vi "UHR-Fleezers Control (host) - 11.1.vi"() -> ()   [LabVIEW 2012] (continued)
            n2044 = Unbundle By Name(w3406) -> ("Set 1"=w3405:dbl, "Set 2"=w3404:dbl)
            n2045 = Unbundle By Name(w3412) -> ("Set 1"=w3411:dbl, "Set 2"=w3410:dbl)
            n2046 = Unbundle By Name(w3409) -> ("Set 1"=w3408:bool, "Set 2"=w3407:bool)
            n2047 = Select(t=w3405, s=w3408, f=w3411) -> (s? t:f=w3403:dbl)
            n2048 = Select(t=w3404, s=w3407, f=w3410) -> (s? t:f=w3402:dbl)
            n2049 = Bundle By Name(cluster=w3412, "Set 1"=w3403, "Set 2"=w3402) -> (w3400:cluster{"Set 1":dbl, "Set 2":dbl})
            n2050 = local write "Setpoints (V)"(w3400) -> ()
            n2051 = Multiply(x=3276.7, y=w3400) -> (x*y=w3401:cluster{"Set 1":dbl, "Set 2":dbl})
            n2052 = To Word Integer(number=w3401) -> (16bit integer=w3413:cluster{"Set 1":i16, "Set 2":i16})
          }
        }
        n2053 = Unbundle By Name(w3385) -> ("Set 1"=w3384:i16, "Set 2"=w3383:i16)
        n2054 = xnode "Read/Write Control"("FPGA VI Reference In"=w3381, "error in"=w3380, "FB Setpoint Set 1"=w3384, "FB Setpoint Set 2"=w3383) -> ("error out"=w3379:errorcluster)  [unwired: 1 out]
      }
      event "Invert GI": Value Change {
        n2055 = event-data() -> ()  [unwired: 7 out]
        n2056 = xnode "Read/Write Control"("FPGA VI Reference In"=w3418, "error in"=w3416, "Invert GI"="Invert GI", "Invert GI 2"="Invert GI") -> ("error out"=w3417:errorcluster)  [unwired: 1 out]
      }
      event "Green FB Setpoint (mV)", "Green FB Gains", "Green FB On/Off", "Current When FB OFF (%)", "Green int current ON count adj": Value Change {
        n2057 = event-data() -> ()  [unwired: 7 out]
        n2058 = local read "Green FB Setpoint (mV)"() -> (w3425:dbl)
        n2059 = local read "Current When FB OFF (%)"() -> (w3428:dbl)
        n2060 = Multiply(x=w3425, y=3.2767) -> (x*y=w3424:dbl)
        n2061 = Multiply(x=w3428, y=655.35) -> (x*y=w3429:dbl)
        n2062 = To Unsigned Word Integer(number=w3429) -> (unsigned 16bit integer=w3427:u16)
        n2063 = local read "Green int current ON count adj"() -> (w3432:u32)
        n2064 = local read "Green FB Gains"() -> (w3431:T14)
        n2065 = local read "Green Laser ON/Interlacing"() -> (w3422:bool)
        n2066 = local read "Green laser mode"() -> (w3421:enum32{"Laser ON", "Laser OFF", "Interlace"})
        n2067 = local read "Green FB On/Off"() -> (w3433:bool)
        n2068 = Equal?(x=w3421, y=enum32{"Laser ON", "Laser OFF", "Interlace"}."Interlace") -> (x = y?=w3419:bool)
        n2069 = Compound Arithmetic op=AND(w3419, w3433, w3422) -> (w3423:bool)
        n2070 = xnode "Read/Write Control"("FPGA VI Reference In"=w3436, "error in"=w3435, "Green FB Setpoint"=w3424, "Green FB On/Off"=w3423, "Current Out"=w3427, "Green int current ON count adj"=w3432, "Green FB Gains"=w3431) -> ("error out"=w3434:errorcluster)  [unwired: 1 out]
      }
      event "Green laser mode", "Green Laser ON/Interlacing": Value Change {
        n2071 = event-data() -> ()  [unwired: 7 out]
        n2072 = local write "Green Laser ON/OFF"("Green Laser ON/Interlacing") -> ()
        n2073 = case shown="True" "Green Laser ON/Interlacing" {
          tunnel: "Green laser mode" -> [_ w3450]
          tunnel: [enum32{"Laser ON", "Laser OFF", "Interlace"}."Laser OFF" ("Green laser mode") w3450] -> w3439
          tunnel: [FALSE w3446] -> w3438
          frame False {
          }
          frame True {
            n2074 = local read "Green FB On/Off"() -> (w3447:bool)
            n2075 = Equal?(x=w3450, y=enum32{"Laser ON", "Laser OFF", "Interlace"}."Interlace") -> (x = y?=w3448:bool)
            n2076 = And(x=w3448, y=w3447) -> (x .and. y?=w3446:bool)
          }
        }
        n2077 = xnode "Read/Write Control"("FPGA VI Reference In"=w3443, "error in"=w3441, "Operating Mode"=w3439, "Operating Mode 2"=w3439, "Green FB On/Off"=w3438) -> ("error out"=w3442:errorcluster)  [unwired: 1 out]
      }
      event "Green Laser ON/OFF": Value Change {
        n2078 = event-data() -> ()  [unwired: 7 out]
        n2079 = property on="Green Laser ON/Interlacing" class="Bool (strict)"("Val(Sgnl)"="Green Laser ON/OFF") -> ()  [unwired: 2 in, 2 out]
      }
      event "Test ttrig": Value Change {
        n2080 = event-data() -> ()  [unwired: 7 out]
        n2081 = xnode "Read/Write Control"("FPGA VI Reference In"=w3455, "error in"=w3454, "TTrig?"=TRUE) -> ("error out"=w3453:errorcluster)  [unwired: 1 out]
      }
      event "Neg. TTrig FPGA": Value Change {
        n2082 = event-data() -> ()  [unwired: 7 out]
        n2083 = xnode "Read/Write Control"("FPGA VI Reference In"=w3459, "error in"=w3458, "TTrig Negate Pos"="Neg. TTrig FPGA") -> ()  [unwired: 2 out]
      }
      event "- phase (APD 1 Gate)", "+ phase (APD 1 Gate)": Value Change {
        n2084 = event-data() -> ()  [unwired: 7 out]
        n2085 = local read "Phase Adj. (APD 1 Gate)"() -> (w3460:i16)
        n2086 = Negate(x=w3460) -> (-x=w3468:i16)
        n2087 = Select(t=w3468, s="- phase (APD 1 Gate)", f=w3460) -> (s? t:f=w3467:i16)
        n2088 = Or(x="- phase (APD 1 Gate)", y="+ phase (APD 1 Gate)") -> (x .or. y?=w3463:bool)
        n2089 = xnode "Read/Write Control"("FPGA VI Reference In"=w3470, "error in"=w3469, "Phase count adjustment (APD 1 Gate)"=w3467) -> ("FPGA VI Reference Out"=w3465:T19, "error out"=w3466:errorcluster)
        n2090 = xnode "Read/Write Control"("FPGA VI Reference In"=w3465, "error in"=w3466, "+ phase (APD 1 Gate)"=w3463) -> ("error out"=w3464:errorcluster)  [unwired: 1 out]
      }
      event "+ phase (APD 2 Gate)", "- phase (APD 2 Gate)": Value Change {
        n2091 = event-data() -> ()  [unwired: 7 out]
        n2092 = local read "Phase Adj. (APD 2 Gate)"() -> (w3471:i16)
        n2093 = Negate(x=w3471) -> (-x=w3479:i16)
        n2094 = Select(t=w3479, s="- phase (APD 2 Gate)", f=w3471) -> (s? t:f=w3478:i16)
        n2095 = Or(x="- phase (APD 2 Gate)", y="+ phase (APD 2 Gate)") -> (x .or. y?=w3474:bool)
        n2096 = xnode "Read/Write Control"("FPGA VI Reference In"=w3481, "error in"=w3480, "Phase count adjustment (APD 2 Gate)"=w3478) -> ("FPGA VI Reference Out"=w3476:T19, "error out"=w3477:errorcluster)
        n2097 = xnode "Read/Write Control"("FPGA VI Reference In"=w3476, "error in"=w3477, "+ phase (APD 2 Gate)"=w3474) -> ("error out"=w3475:errorcluster)  [unwired: 1 out]
      }
      event "Phase Adj. (APD Acq)", "+ phase (APD Acq)", "- phase (APD Acq)": Value Change {
        n2098 = event-data() -> ()  [unwired: 7 out]
        n2099 = local read "Phase Adj. (APD Acq)"() -> (w3484:i16)
        n2100 = Negate(x=w3484) -> (-x=w3490:i16)
        n2101 = Select(t=w3490, s="+ phase (APD Acq)", f=w3484) -> (s? t:f=w3489:i16)
        n2102 = Or(x="+ phase (APD Acq)", y="- phase (APD Acq)") -> (x .or. y?=w3485:bool)
        n2103 = xnode "Read/Write Control"("FPGA VI Reference In"=w3492, "error in"=w3491, "Phase Count Adjustment (APD Acq)"=w3489) -> ("FPGA VI Reference Out"=w3487:T19, "error out"=w3488:errorcluster)
        n2104 = xnode "Read/Write Control"("FPGA VI Reference In"=w3487, "error in"=w3488, "+ phase (APD Acq)"=w3485) -> ("error out"=w3486:errorcluster)  [unwired: 1 out]
      }
      event "Phase adj. (GI)", "+ phase (GI)", "- phase (GI)": Value Change {
        n2105 = event-data() -> ()  [unwired: 7 out]
        n2106 = Negate(x="Phase adj. (GI)") -> (-x=w3501:i16)
        n2107 = Select(t=w3501, s="+ phase (GI)", f="Phase adj. (GI)") -> (s? t:f=w3500:i16)
        n2108 = Or(x="+ phase (GI)", y="- phase (GI)") -> (x .or. y?=w3496:bool)
        n2109 = xnode "Read/Write Control"("FPGA VI Reference In"=w3503, "error in"=w3502, "Phase count adjustment (GI)"=w3500) -> ("FPGA VI Reference Out"=w3498:T19, "error out"=w3499:errorcluster)
        n2110 = xnode "Read/Write Control"("FPGA VI Reference In"=w3498, "error in"=w3499, "+ phase (GI)"=w3496) -> ("error out"=w3497:errorcluster)  [unwired: 1 out]
      }
      event "Phase adj. (GI) 2", "+ phase (GI) 2", "- phase (GI) 2": Value Change {
        n2111 = event-data() -> ()  [unwired: 7 out]
        n2112 = Negate(x="Phase adj. (GI) 2") -> (-x=w3512:i16)
        n2113 = Select(t=w3512, s="+ phase (GI) 2", f="Phase adj. (GI) 2") -> (s? t:f=w3511:i16)
        n2114 = Or(x="+ phase (GI) 2", y="- phase (GI) 2") -> (x .or. y?=w3507:bool)
        n2115 = xnode "Read/Write Control"("FPGA VI Reference In"=w3514, "error in"=w3513, "Phase count adjustment (GI) 2"=w3511) -> ("FPGA VI Reference Out"=w3509:T19, "error out"=w3510:errorcluster)
        n2116 = xnode "Read/Write Control"("FPGA VI Reference In"=w3509, "error in"=w3510, "+ phase (GI) 2"=w3507) -> ("error out"=w3508:errorcluster)  [unwired: 1 out]
      }
      event "Phase adj. (Green FB)", "- phase (Green FB)", "+ phase (Green FB)": Value Change {
        n2117 = event-data() -> ()  [unwired: 7 out]
        n2118 = Negate(x="Phase adj. (Green FB)") -> (-x=w3523:i16)
        n2119 = Select(t=w3523, s="+ phase (Green FB)", f="Phase adj. (Green FB)") -> (s? t:f=w3522:i16)
        n2120 = Or(x="+ phase (Green FB)", y="- phase (Green FB)") -> (x .or. y?=w3518:bool)
        n2121 = xnode "Read/Write Control"("FPGA VI Reference In"=w3525, "error in"=w3524, "Phase count adjustment (Green FB)"=w3522) -> ("FPGA VI Reference Out"=w3520:T19, "error out"=w3521:errorcluster)
        n2122 = xnode "Read/Write Control"("FPGA VI Reference In"=w3520, "error in"=w3521, "+ phase (Green FB)"=w3518) -> ("error out"=w3519:errorcluster)  [unwired: 1 out]
      }
      event "Invert APD Gate", "APD Gate ON Count", "APD Gate OFF Count", "APD Gate", "APD Integration Time (s)", "APD 1 AO Mult.", "APD 2 AO Mult.", "On one out of X cycles": Value Change {
        n2123 = event-data() -> ()  [unwired: 7 out]
        n2124 = Add(x="GI Frequency, ON count", y="GI Frequency, OFF count") -> (x+y=w3529:u32)
        n2125 = Add(x="APD Gate ON Count", y="APD Gate OFF Count") -> (x+y=w3542:u32)
        n2126 = Multiply(x="On one out of X cycles", y=w3529) -> (x*y=w3526:u32)
        "Green FB Count" <- w3526
        n2127 = Subtract(x=w3526, y="GI Frequency, ON count") -> (x-y=w3527:u32)
        n2128 = Multiply(x=w3542, y="On one out of X cycles") -> (x*y=w3541:u32)
        n2129 = Subtract(x=w3541, y="APD Gate ON Count") -> (x-y=w3540:u32)
        n2130 = local read "DMA Update Period (s)"() -> (w3543:dbl)
        n2131 = Multiply(x="APD Integration Time (s)", y=40000000.0) -> (x*y=w3548:dbl)
        n2132 = Reciprocal(x="APD Integration Time (s)") -> (1/x=→"APD Acq Rate (Hz)":dbl)
        n2133 = To Unsigned Long Integer(number=w3548) -> (unsigned 32bit integer=w3532:u32)
        "APD Int. Count" <- w3532
        n2134 = xnode "Read/Write Control"("FPGA VI Reference In"=w3552, "error in"=w3551, "Invert APD Gate"="Invert APD Gate", "APD Gate ON Count"="APD Gate ON Count", "APD Gate OFF Count"=w3540, "APD Acq Rate Count"=w3532, "APD Gate Operating Mode"="APD Gate", "APD 1 AO scale factor"="APD 1 AO Mult.", "APD 2 AO scale factor"="APD 2 AO Mult.", "Green interlace ON count"="GI Frequency, ON count", "Green interlace OFF count"=w3527, "Green interlace ON count 2"="GI Frequency, ON count", "Green interlace OFF count 2"=w3527, "Green FB Count"=w3526) -> ("error out"=w3550:errorcluster)  [unwired: 1 out]
        n2135 = Divide(x=w3543, y="APD Integration Time (s)") -> (x/y=w3546:dbl)
        n2136 = Multiply(x=2.0, y=w3546) -> (x*y=w3545:dbl)
        n2137 = local write "APD Samples/FIFO Acq."(w3546) -> ()
        n2138 = local write "APD Elements/DMA read"(w3545) -> ()
      }
      event "Number of F/B Scans (AOD)", "Scan Speed (nm/s)", "Scan BD", "Initial delta (MHz)", "Step Size (nm)", "Scan Range (nm)": Value Change {
        w3614 = 123.0  # AOM cal (nm/MHz)
        n2139 = event-data() -> ()  [unwired: 7 out]
        n2140 = local read "BD 1 Frequency 1 (MHz)"() -> (w3597:dbl)
        n2141 = local read "AOM X Cal (nm/MHz)"() -> (w3589:dbl)
        n2142 = local read "X RF Frequency Limits (MHz)"() -> (w3601:T16)
        n2143 = local read "Y RF Frequency Limits (MHz)"() -> (w3598:T16)
        n2144 = local read "BD 2 Frequency 1 (MHz)"() -> (w3603:dbl)
        n2145 = Negate(x="Scan Range (nm)") -> (-x=w3567:dbl)
        n2146 = Divide(x=w3567, y=w3589) -> (x/y=w3571:dbl)
        n2147 = Select(t=w3601, s="Scan BD", f=w3598) -> (s? t:f=w3600:T16)
        n2148 = Select(t=w3597, s="Scan BD", f=w3603) -> (s? t:f=w3602:dbl)
        n2149 = Unbundle By Name(w3600) -> ("Maximum"=w3609:dbl, "Minimum"=w3608:dbl)
        n2150 = Add(x=w3571, y=w3602) -> (x+y=w3606:dbl)
        n2151 = Divide(x=w3567, y="Step Size (nm)") -> (x/y=w3586:dbl)
        n2152 = Divide(x="Step Size (nm)", y=w3589) -> (x/y=w3595:dbl)
        n2153 = Absolute Value(x=w3586) -> (abs(x)=w3570:dbl)
        n2154 = Sign(1:w3567) -> (0:w3568:dbl)
        n2155 = In Range and Coerce(upper limit=w3609, x=w3606, lower limit=w3608) -> (coerced(x)=w3605:dbl, In Range?=w3607:bool)
        n2156 = To Unsigned Quad Integer(1:w3570) -> (0:w3585:u64)
        "Scan steps (AOD)" <- w3585
        n2157 = call "IR AOM freq to word.vi"("Frequency In (MHz)"=w3595) -> ("Frequency Word Out (double)"=w3592:dbl)
        n2158 = Multiply(x=w3568, y=w3592) -> (x*y=w3569:dbl)
        n2159 = Subtract(x=w3606, y=w3605) -> (x-y=w3604:dbl)
        n2160 = To Quad Integer(1:w3569) -> (0:w3591:i64)
        "Incr. int (AOD)" <- w3591
        n2161 = Subtract(x=w3571, y=w3604) -> (x-y=w3590:dbl)
        "Scan Range (MHz)" <- w3590
        n2162 = Select(t=w3571, s=w3607, f=w3590) -> (s? t:f=w3610:dbl)
        n2163 = Multiply(x=w3590, y=w3589) -> (x*y=w3588:dbl)
        n2164 = Decrement(x=w3585) -> (x-1=w3638:u64)
        n2165 = Negate(x=w3588) -> (-x=w3584:dbl)
        n2166 = local write "Scan Range (nm)"(w3584) -> ()
        n2167 = Divide(x=w3610, y=w3638) -> (x/y=w3594:dbl)
        "Scan Increment (MHz)" <- w3594
        n2168 = call "IR AOM freq to word.vi"("Frequency In (MHz)"=w3594) -> ("Frequency Word Out (double)"=w3593:dbl)
        n2169 = Divide(x="Step Size (nm)", y="Scan Speed (nm/s)") -> (x/y=w3581:dbl)
        n2170 = To Quad Integer(1:w3593) -> ()  [unwired: 1 out]
        n2171 = local read "Number Interlace Sets"() -> (w3565:u8)
        n2172 = local read "AI Count (ticks)"() -> (w3566:u32)
        n2173 = local read "Total Counts (ticks)"() -> (w3564:u32)
        n2174 = local read "# Samples/trap"() -> (w3596:u32)
        n2175 = Multiply(x=w3566, y=w3565) -> (x*y=w3563:u32)
        n2176 = Divide(x=w3564, y=w3563) -> (x/y=w3562:dbl)
        n2177 = Select(t=w3597, s="Scan BD", f=w3603) -> (s? t:f=w3635:dbl)
        "Initial freq. (MHz)" <- w3635
        n2178 = Add(x=w3610, y=w3635) -> (x+y=→"Final freq. (MHz)":dbl)
        n2179 = Divide(x=w3564, y=40000000.0) -> (x/y=w3580:dbl)
        n2180 = Divide(x=w3581, y=w3580) -> (x/y=w3579:dbl)
        n2181 = To Unsigned Quad Integer(1:w3579) -> (0:w3554:u64)
        n2182 = Quotient & Remainder(x=w3554, y=u64 2) -> (x-y*floor(x/y)=w3558:u64)  [unwired: 1 out]
        n2183 = Equal?(x=w3558, y=u64 0) -> (x = y?=w3556:bool)
        n2184 = Decrement(x=w3554) -> (x-1=w3555:u64)
        n2185 = Select(t=w3554, s=w3556, f=w3555) -> (s? t:f=w3553:u64)
        "Cycles/step (AOD)" <- w3553
        n2186 = xnode "Read/Write Control"("FPGA VI Reference In"=w3646, "error in"=w3645, "Scan steps"=w3585, "Number of scans"="Number of F/B Scans (AOD)", "Cycles per step"=w3553, "Scan freq.  increment"=w3591, "Scan BD"="Scan BD") -> ("error out"=w3644:errorcluster)  [unwired: 1 out]
        n2187 = Multiply(x=w3585, y=w3553) -> (x*y=w3639:u64)
        n2188 = Multiply(x=w3639, y=u64 2) -> (x*y=w3561:u64)
        n2189 = Multiply(x=w3562, y=w3561) -> (x*y=w3560:dbl)
        "Data points/scan (f/b)" <- w3560
        n2190 = Multiply(x=w3560, y="Number of F/B Scans (AOD)") -> (x*y=w3642:dbl)
        "Data points/scans" <- w3642
        n2191 = Divide(x=w3642, y=w3596) -> (x/y=→"N sets should be saved":dbl)
        n2192 = Multiply(x=w3639, y=w3580) -> (x*y=w3578:dbl)
        "Time/Scan (s) (AOD)" <- w3578
        n2193 = Select(t=w3610, s="Scan BD", f=0.0) -> (s? t:f=w3636:dbl)
        n2194 = Select(t=0.0, s="Scan BD", f=w3610) -> (s? t:f=w3632:dbl)
        n2195 = local read "BD 2 Frequency 2 (MHz)"() -> (w3628:dbl)
        n2196 = local read "BD 1 Frequency 2 (MHz)"() -> (w3631:dbl)
        n2197 = Add(x=w3632, y=w3603) -> (x+y=w3629:dbl)
        n2198 = Add(x=w3597, y=w3636) -> (x+y=w3630:dbl)
        n2199 = Multiply(x=w3578, y=2.0) -> (x*y=w3577:dbl)
        n2200 = Multiply(x=w3577, y="Number of F/B Scans (AOD)") -> (x*y=w3574:dbl)
        n2201 = Divide(x=w3574, y=60.0) -> (x/y=→"Time to Finish All (min)":dbl)
        n2202 = Add(x="Trap 2 Bead Size (nm)", y="Trap 1 Bead Size (nm)") -> (x+y=w3618:dbl)
        n2203 = Divide(x=w3618, y=2.0) -> (x/y=w3612:dbl)
        n2204 = local read "Initial delta (MHz)"() -> (w3615:dbl)
        n2205 = Subtract(x=w3629, y=w3628) -> (x-y=w3626:dbl)
        n2206 = Subtract(x=w3630, y=w3631) -> (x-y=w3627:dbl)
        n2207 = Square(x=w3626) -> (x^2=w3625:dbl)
        n2208 = Square(x=w3627) -> (x^2=w3624:dbl)
        n2209 = Add(x=w3624, y=w3625) -> (x+y=w3623:dbl)
        n2210 = Square Root(x=w3623) -> (sqrt(x)=w3622:dbl)
        "Final delta (MHz)" <- w3622
        n2211 = Multiply(x=w3614, y=w3622) -> (x*y=w3621:dbl)
        n2212 = Multiply(x=w3615, y=w3614) -> (x*y=w3613:dbl)
        n2213 = Subtract(x=w3613, y=w3612) -> (x-y=→"Initial sep (nm)":dbl)
        n2214 = Subtract(x=w3621, y=w3612) -> (x-y=→"Final sep (nm)":dbl)
      }
      event "Freq or Amp switch first", "Swap F1 and F2", "Freq switch delay", "Amp switch delay": Value Change {
        n2215 = event-data() -> ()  [unwired: 7 out]
        n2216 = local read "Freq or Amp switch first"() -> (w3647:bool)
        n2217 = local read "Amp switch delay"() -> (w3648:u16)
        n2218 = local read "Freq switch delay"() -> (w3650:u16)
        n2219 = local read "Swap F1 and F2"() -> (w3649:bool)
        n2220 = xnode "Read/Write Control"("FPGA VI Reference In"=w3653, "error in"=w3652, "Freq switch delay"=w3650, "Swap F1 and F2"=w3649, "Amp switch delay"=w3648, "Freq or Amp switch first"=w3647) -> ("error out"=w3651:errorcluster)  [unwired: 1 out]
      }
      event "Scan steps (MCL)", "Number of scans (MCL)", "Scan Range (V)\n(of steps)", "2D or 1D Scan", "N APD Samp/step", "Fast Scan Dir", "Continuous MCL Scanning", "Scan lines (y)": Value Change {
        w3655 = 32767.0 ("y")
        n2221 = event-data() -> ()  [unwired: 7 out]
        n2222 = Select(t="Scan lines (y)", s="2D or 1D Scan", f="Number of scans (MCL)") -> (s? t:f=w3660:u64)
        n2223 = Decrement(x="Scan steps (MCL)") -> (x-1=w3676:u64)
        n2224 = Divide(x="Scan Range (V)\n(of steps)", y=w3676) -> (x/y=w3675:dbl)
        "Desired Scan Incr (V)" <- w3675
        n2225 = local read "APD Integration Time (s)"() -> (w3668:dbl)
        n2226 = Multiply(x=w3675, y=w3655) -> (x*y=w3684:dbl)
        n2227 = Divide(x=w3684, y=10.0) -> (x/y=w3674:dbl)
        "Desired incr (int)" <- w3674
        n2228 = local read "Update Count (MCL)"() -> (w3680:u32)
        n2229 = Round Toward -Infinity(1:w3674) -> (0:w3683:dbl)
        n2230 = To Word Integer(number=w3683) -> (16bit integer=w3658:i16)
        "Actual Incr. int (MCL)" <- w3658
        n2231 = Multiply(x=w3668, y=40000000.0) -> (x*y=w3681:dbl)
        n2232 = Divide(x=w3681, y=w3680) -> (x/y=w3679:dbl)
        n2233 = Multiply(x=i16 10, y=w3658) -> (x*y=w3656:i16)
        n2234 = Multiply(x="N APD Samp/step", y=w3679) -> (x*y=w3678:dbl)
        "Cycles/step (MCL)" <- w3678
        n2235 = Divide(x=w3656, y=w3655) -> (x/y=→"Actual MCL Inc (V)":dbl)
        n2236 = Multiply(x="N APD Samp/step", y="Scan steps (MCL)") -> (x*y=w3670:dbl)
        n2237 = local read "APD Samples/FIFO Acq."() -> (w3667:dbl)
        n2238 = Multiply(x=w3670, y=u64 2) -> (x*y=w3669:dbl)
        "Data points/scan (f+b)" <- w3669
        n2239 = Multiply(x=w3669, y=w3660) -> (x*y=w3687:dbl)
        "Data points/scans (MCL)" <- w3687
        n2240 = Multiply(x=w3668, y=w3669) -> (x*y=w3661:dbl)
        "Time/f+b scan (s) (MCL)" <- w3661
        n2241 = Divide(x=w3687, y=w3667) -> (x/y=→"N sets should be saved (MCL)":dbl)
        n2242 = Multiply(x=w3661, y=w3660) -> (x*y=→"Total Time (s)":dbl)
        n2243 = Not(x="Fast Scan Dir") -> (.not. x?=w3665:bool)
        n2244 = xnode "Read/Write Control"("FPGA VI Reference In"=w3691, "error in"=w3690, "Scan steps (MCL)"="Scan steps (MCL)", "Number of scans (MCL)"=w3660, "Cycles per step (MCL)"=w3678, "Scan freq.  increment (MCL)"=w3658, "1D or 2D Scan?"="2D or 1D Scan", "MCL Scan Axis"=w3665, "Cont. Scan (MCL)"="Continuous MCL Scanning") -> ("error out"=w3689:errorcluster)  [unwired: 1 out]
      }
      event "Read Cal": Value Change {
        w3693 = 1000.0 ("y")
        n2245 = event-data() -> ()  [unwired: 7 out]
        n2246 = local read "Save file name"() -> (w3718:path)
        n2247 = local write "Read Cal"(FALSE ("Read Cal")) -> ()
        n2248 = Strip Path(path=w3718) -> (stripped path=w3717:path)  [unwired: 1 out]
        n2249 = Path To String(path=w3717) -> (string=w3716:string)
        n2250 = Concatenate Strings(w3716, "\\current.cal" ("string")) -> (w3714:string)
        n2251 = String To Path(string=w3714) -> (path=w3713:path)
        n2252 = Open/Create/Replace File(file path (use dialog)=w3713, operation (0:open)=T35."open", access (0:read/write)=enum16{"read/write", "read-only", "write-only"}."read-only") -> (refnum out=w3721:refnum<file>, error out=w3707:errorcluster)  [unwired: 1 in, 3 out]
        n2253 = Deny Access(4:w3707, 7:w3721) -> (0:w3706:errorcluster, 3:w3712:refnum<file>)  [unwired: 1 out]
        n2254 = Read from Binary File(5:0.0, 8:w3706, 9:T36."big-endian, network order" ("byte order (0:big-endian, network order)"), 10:-1 ("count (1)"), 11:w3712) -> (0:w3705:errorcluster, 2:w3703:dbl[], 3:w3708:refnum<file>)  [unwired: 2 out]
        n2255 = Array To Cluster(array=w3703) -> (cluster=w3702:T46)
        n2256 = Unbundle(w3702) -> ("[0]"=w3701:dbl, "[1]"=w3700:dbl, "[2]"=w3699:dbl, "[3]"=w3698:dbl, "[4]"=w3697:dbl, "[5]"=w3696:dbl)
        n2257 = Close File(refnum=w3708, error in=w3705) -> (error out=→"Read cal error":errorcluster)  [unwired: 1 out]
        n2258 = Multiply(x=w3696, y=w3693) -> (x*y=w3694:dbl)
        n2259 = local write "T2 kappa_x (pN/nm)"(w3698) -> ()
        n2260 = local write "T1 kappa_x (pN/nm)"(w3699) -> ()
        n2261 = local write "T1 alpha_x (nm/V)"(w3701) -> ()
        n2262 = local write "T2 alpha_x (nm/V)"(w3700) -> ()
        n2263 = Multiply(x=w3697, y=w3693) -> (x*y=w3695:dbl)
        n2264 = local write "T1 offset_x (mV)"(w3695) -> ()
        n2265 = local write "T2 offset_x (mV)"(w3694) -> ()
      }
      event "Abort MCL Scan": Value Change {
        n2266 = event-data() -> ()  [unwired: 7 out]
        n2267 = local write "MCL Scanning"(FALSE ("MCL Scanning")) -> ()
        n2268 = xnode "Read/Write Control"("FPGA VI Reference In"=w3726, "error in"=w3725, "Abort scan (MCL)"="Abort MCL Scan") -> ("error out"=w3724:errorcluster)  [unwired: 1 out]
      }
      event "Update Count (MCL)": Value Change {
        n2269 = event-data() -> ()  [unwired: 7 out]
        n2270 = xnode "Read/Write Control"("FPGA VI Reference In"=w3730, "error in"=w3729, "MCL count"="Update Count (MCL)") -> ("error out"=w3728:errorcluster)  [unwired: 1 out]
      }
      event "Phase adjust (MCL)", "+ phase (MCL)", "- phase (MCL)": Value Change {
        n2271 = event-data() -> ()  [unwired: 7 out]
        n2272 = Negate(x="Phase adjust (MCL)") -> (-x=w3739:i16)
        n2273 = Select(t=w3739, s="- phase (MCL)", f="Phase adjust (MCL)") -> (s? t:f=w3737:i16)
        n2274 = Or(x="- phase (MCL)", y="+ phase (MCL)") -> (x .or. y?=w3732:bool)
        n2275 = xnode "Read/Write Control"("FPGA VI Reference In"=w3741, "error in"=w3740, "Phase count adjustment (MCL)"=w3737) -> ("FPGA VI Reference Out"=w3733:T19, "error out"=w3734:errorcluster)
        n2276 = xnode "Read/Write Control"("FPGA VI Reference In"=w3733, "error in"=w3734, "+ phase (MCL)"=w3732) -> ("error out"=w3731:errorcluster)  [unwired: 1 out]
      }
      event "Abort AOD Scan": Value Change {
        n2277 = event-data() -> ()  [unwired: 7 out]
        n2278 = xnode "Read/Write Control"("FPGA VI Reference In"=w3745, "error in"=w3744, "Abort scan"="Abort AOD Scan") -> ("error out"=w3743:errorcluster)  [unwired: 1 out]
      }
      event "Continuous AOD Scanning": Value Change {
        n2279 = event-data() -> ()  [unwired: 7 out]
        n2280 = xnode "Read/Write Control"("FPGA VI Reference In"=w3749, "error in"=w3748, "Cont. Scan"="Continuous AOD Scanning") -> ("error out"=w3747:errorcluster)  [unwired: 1 out]
      }
      event "Index": Value Change {
        n2281 = event-data() -> ()  [unwired: 7 out]
        n2282 = call "Create new save file.vi"("Insert"="", "Ext"=".dat" ("string"), "Index In"="Index") -> ("Path Out"=→"Save file name":path, "Index Out"=w3750:dbl)
        "Save index" <- w3750
        n2283 = local write "Index"(w3750) -> ()
      }
      event "AO1", "AO2": Value Change {
        w3765 = 10.0 ("y")
        w3764 = 32767.0 ("y")
        n2284 = event-data() -> ()  [unwired: 7 out]
        n2285 = local read "AO2"() -> (w3763:dbl)
        n2286 = local read "AO1"() -> (w3760:dbl)
        n2287 = Multiply(x=w3760, y=w3764) -> (x*y=w3759:dbl)
        n2288 = Multiply(x=w3763, y=w3764) -> (x*y=w3762:dbl)
        n2289 = Divide(x=w3759, y=w3765) -> (x/y=w3758:dbl)
        n2290 = Divide(x=w3762, y=w3765) -> (x/y=w3761:dbl)
        n2291 = To Word Integer(number=w3758) -> (16bit integer=w3766:i16)
        n2292 = To Word Integer(number=w3761) -> (16bit integer=w3767:i16)
        n2293 = xnode "Read/Write Control"("FPGA VI Reference In"=w3757, "error in"=w3756, "AO1"=w3766, "AO2"=w3767) -> ("error out"=w3755:errorcluster)  [unwired: 1 out]
      }
      event "Inject Pump 1": Value Change {
        n2294 = event-data() -> ()  [unwired: 7 out]
        n2295 = local read "Use Harvard pumps\nfor beads (else Chemyx)"() -> (w3769:bool)
        n2296 = case shown="True" w3769 {
          tunnel: "Inject Pump 1" -> [w3773 w3811]
          tunnel: w3768 -> [_ w3812]
          frame False {
            n2297 = local read "Pump write delay (ms)"() -> (w3772:dbl)
            n2298 = local read "Chemyx Syringe Pump Serial Port"() -> (w3771:refnum<visa-resource-name>)
            n2299 = case shown="True" w3773 {
              tunnel: w3772 -> [w3779 w3793]
              tunnel: w3771 -> [w3776 w3792]
              frame False {
                n2300 = flat-sequence {
                  tunnel: w3776 -> [w3780]
                  tunnel: [w3780] -> w3777
                  tunnel: w3779 -> [_]
                  tunnel: [w3783] -> w3778
                  tunnel: w3777 -> [w3783]
                  tunnel: w3778 -> [w3784]
                  tunnel: [w3784] -> w3774
                  tunnel: [w3786] -> w3775
                  tunnel: w3774 -> [w3786]
                  tunnel: w3775 -> [w3788]
                  frame #0 {
                    n2301 = call "Write to pump.vi"("string"="enter pump1", "VISA resource name"=w3780) -> ()  [unwired: 1 out]
                  }
                  frame #1 {
                    n2302 = Wait (ms)(milliseconds to wait="Pump pause delay (ms)") -> ()  [unwired: 1 out]
                  }
                  frame #2 {
                    n2303 = call "Write to pump.vi"("string"="stop", "VISA resource name"=w3784) -> ()  [unwired: 1 out]
                  }
                  frame #3 {
                    n2304 = Wait (ms)(milliseconds to wait=u32 500) -> ()  [unwired: 1 out]
                  }
                  frame #4 {
                    n2305 = call "Write to pump.vi"("string"="stop", "VISA resource name"=w3788) -> ()  [unwired: 1 out]
                  }
                }
              }
              frame True {
                n2306 = flat-sequence {
                  tunnel: w3792 -> [w3802]
                  tunnel: w3793 -> [w3797]
                  tunnel: w3793 -> [w3804]
                  tunnel: w3792 -> [w3805]
                  tunnel: [w3805] -> w3790
                  tunnel: [w3807] -> w3791
                  tunnel: w3790 -> [w3807]
                  tunnel: w3791 -> [w3809]
                  frame #0 {
                    n2307 = local read "All Pump Parameters"() -> (w3796:T5)
                    n2308 = Unbundle By Name(w3796) -> ("Pump 1"=w3803:T47)
                    n2309 = call "Set pump parameters.vi"("Pump write delay (ms)"=w3797, "Volume (uL)"="Ch 1 Inject Volume (uL)", "Rate (uL/h)"="Ch 1 Inject Rate (ul/h)", "Units"=4.0, "Pump #"=1.0, "Pump Parameters In"=w3803, "VISA resource name"=w3802) -> ("Pump Parameters Out"=w3795:T47)  [unwired: 3 in]
                    n2310 = Bundle By Name(cluster=w3796, "Pump 1"=w3795) -> (w3794:T5)
                    n2311 = local write "All Pump Parameters"(w3794) -> ()
                  }
                  frame #1 {
                    n2312 = Wait (ms)(milliseconds to wait=w3804) -> ()  [unwired: 1 out]
                  }
                  frame #2 {
                    n2313 = call "Write to pump.vi"("string"="start", "VISA resource name"=w3805) -> ()  [unwired: 1 out]
                  }
                  frame #3 {
                    n2314 = Wait (ms)(milliseconds to wait=u32 500) -> ()  [unwired: 1 out]
                  }
                  frame #4 {
                    n2315 = call "Write to pump.vi"("string"="start", "VISA resource name"=w3809) -> ()  [unwired: 1 out]
                  }
                }
              }
            }
          }
          frame True {
            n2316 = case shown="False" w3811 {
              tunnel: w3812 -> [w3813 w3823]
              frame False {
                n2317 = flat-sequence {
                  tunnel: w3813 -> [w3815]
                  frame #0 {
                    n2318 = local write "Flushing P1"(FALSE ("Flushing P1")) -> ()
                    n2319 = Concatenate Strings("stop" ("string"), "\r") -> (w3817:string)
                    n2320 = VISA Write(VISA resource name=w3815, write buffer=w3817) -> ()  [unwired: 1 in, 3 out]
                  }
                  frame #1 {
                    n2321 = property on="Clear Volume P1" class="Bool (strict)"("Val(Sgnl)"=TRUE ("Value (Signaling)")) -> ()  [unwired: 2 in, 2 out]
                  }
                }
              }
              frame True {
                n2322 = local read "Normal Flow Rate (ul/h) P1"() -> (w3821:dbl)
                n2323 = Number To Decimal String(number=w3821) -> (decimal integer string=w3827:string)  [unwired: 1 in]
                n2324 = Concatenate Strings("irate  " ("string"), w3827, " u/h" ("string"), "\r") -> (w3825:string)
                n2325 = VISA Write(VISA resource name=w3823, write buffer=w3825) -> (VISA resource name out=w3822:refnum<visa-resource-name>)  [unwired: 1 in, 2 out]
                n2326 = Concatenate Strings("irun" ("string"), "\r") -> (w3829:string)
                n2327 = VISA Write(VISA resource name=w3822, write buffer=w3829) -> ()  [unwired: 1 in, 3 out]
              }
            }
          }
        }
      }
      event "Inject Pump 3": Value Change {
        n2328 = event-data() -> ()  [unwired: 7 out]
        n2329 = local read "Use Harvard pumps\nfor beads (else Chemyx)"() -> (w3832:bool)
        n2330 = case shown="True" w3832 {
          tunnel: "Inject Pump 3" -> [w3836 w3875]
          tunnel: w3831 -> [_ w3874]
          frame False {
            n2331 = local read "Pump write delay (ms)"() -> (w3835:dbl)
            n2332 = case shown="True" w3836 {
              tunnel: w3835 -> [w3842 w3856]
              tunnel: "Chemyx Syringe Pump Serial Port" -> [w3839 w3855]
              frame False {
                n2333 = flat-sequence {
                  tunnel: w3839 -> [w3843]
                  tunnel: [w3843] -> w3840
                  tunnel: w3842 -> [_]
                  tunnel: [w3846] -> w3841
                  tunnel: w3840 -> [w3846]
                  tunnel: w3841 -> [w3847]
                  tunnel: [w3847] -> w3837
                  tunnel: [w3849] -> w3838
                  tunnel: w3837 -> [w3849]
                  tunnel: w3838 -> [w3851]
                  frame #0 {
                    n2334 = call "Write to pump.vi"("string"="enter pump3", "VISA resource name"=w3843) -> ()  [unwired: 1 out]
                  }
                  frame #1 {
                    n2335 = local read "Pump pause delay (ms)"() -> (w3845:u32)
                    n2336 = Wait (ms)(milliseconds to wait=w3845) -> ()  [unwired: 1 out]
                  }
                  frame #2 {
                    n2337 = call "Write to pump.vi"("string"="stop", "VISA resource name"=w3847) -> ()  [unwired: 1 out]
                  }
                  frame #3 {
                    n2338 = Wait (ms)(milliseconds to wait=u32 0) -> ()  [unwired: 1 out]
                  }
                  frame #4 {
                    n2339 = call "Write to pump.vi"("string"="stop", "VISA resource name"=w3851) -> ()  [unwired: 1 out]
                  }
                }
              }
              frame True {
                n2340 = flat-sequence {
                  tunnel: w3855 -> [w3865]
                  tunnel: w3856 -> [w3860]
                  tunnel: w3856 -> [w3867]
                  tunnel: w3855 -> [w3868]
                  tunnel: [w3868] -> w3854
                  tunnel: [w3871] -> w3853
                  tunnel: w3854 -> [w3871]
                  tunnel: w3853 -> [w3872]
                  frame #0 {
                    n2341 = local read "All Pump Parameters"() -> (w3859:T5)
                    n2342 = Unbundle By Name(w3859) -> ("Pump 3"=w3866:T47)
                    n2343 = call "Set pump parameters.vi"("Pump write delay (ms)"=w3860, "Volume (uL)"="Ch 3 Inject Volume (uL)", "Rate (uL/h)"="Ch 3 Inject Rate (ul/h)", "Units"=4.0, "Pump #"=3.0, "Pump Parameters In"=w3866, "VISA resource name"=w3865) -> ("Pump Parameters Out"=w3858:T47)  [unwired: 3 in]
                    n2344 = Bundle By Name(cluster=w3859, "Pump 3"=w3858) -> (w3857:T5)
                    n2345 = local write "All Pump Parameters"(w3857) -> ()
                  }
                  frame #1 {
                    n2346 = Wait (ms)(milliseconds to wait=w3867) -> ()  [unwired: 1 out]
                  }
                  frame #2 {
                    n2347 = call "Write to pump.vi"("string"="start", "VISA resource name"=w3868) -> ()  [unwired: 1 out]
                  }
                  frame #3 {
                    n2348 = Wait (ms)(milliseconds to wait=u32 500) -> ()  [unwired: 1 out]
                  }
                  frame #4 {
                    n2349 = call "Write to pump.vi"("string"="start", "VISA resource name"=w3872) -> ()  [unwired: 1 out]
                  }
                }
              }
            }
          }
          frame True {
            n2350 = case shown="False" w3875 {
              tunnel: w3874 -> [w3876 w3883]
              frame False {
                n2351 = flat-sequence {
                  tunnel: w3876 -> [w3878]
                  frame #0 {
                    n2352 = local write "Flushing P3"(FALSE ("Flushing P3")) -> ()
                    n2353 = Concatenate Strings("stop" ("string"), "\r") -> (w3880:string)
                    n2354 = VISA Write(VISA resource name=w3878, write buffer=w3880) -> ()  [unwired: 1 in, 3 out]
                  }
                  frame #1 {
                    n2355 = property on="Clear Volume P3" class="Bool (strict)"("Val(Sgnl)"=TRUE ("Value (Signaling)")) -> ()  [unwired: 2 in, 2 out]
                  }
                }
              }
              frame True {
                n2356 = local read "Normal Flow Rate (ul/h) P3"() -> (w3884:dbl)
                n2357 = Number To Decimal String(number=w3884) -> (decimal integer string=w3890:string)  [unwired: 1 in]
                n2358 = Concatenate Strings("irate  " ("string"), w3890, " u/h" ("string"), "\r") -> (w3888:string)
                n2359 = VISA Write(VISA resource name=w3883, write buffer=w3888) -> (VISA resource name out=w3886:refnum<visa-resource-name>)  [unwired: 1 in, 2 out]
                n2360 = Concatenate Strings("irun" ("string"), "\r") -> (w3892:string)
                n2361 = VISA Write(VISA resource name=w3886, write buffer=w3892) -> ()  [unwired: 1 in, 3 out]
              }
            }
          }
        }
      }
      event "Inject Pump 2": Value Change {
        n2362 = event-data() -> ()  [unwired: 7 out]
        n2363 = local read "Pump write delay (ms)"() -> (w3896:dbl)
        n2364 = flat-sequence {
          tunnel: w3894 -> [w3909]
          tunnel: w3896 -> [w3905]
          tunnel: "Inject Pump 2" -> [_]
          tunnel: w3896 -> [w3911]
          tunnel: w3894 -> [w3912]
          frame #0 {
            n2365 = local read "All Pump Parameters"() -> (w3904:T5)
            n2366 = Multiply(x=60.0, y="Flush Center Ch Rate (ul/m)") -> (x*y=w3901:dbl)
            n2367 = Unbundle By Name(w3904) -> ("Pump 2"=w3910:T47)
            n2368 = call "Set pump parameters.vi"("Pump write delay (ms)"=w3905, "Volume (uL)"="Flush Center Ch Volume (uL)", "Rate (uL/h)"=w3901, "Units"=3.0, "Pump #"=2.0, "Pump Parameters In"=w3910, "VISA resource name"=w3909) -> ("Pump Parameters Out"=w3903:T47)  [unwired: 3 in]
            n2369 = Bundle By Name(cluster=w3904, "Pump 2"=w3903) -> (w3902:T5)
            n2370 = local write "All Pump Parameters"(w3902) -> ()
            n2371 = Add(x="Flush Center Ch Volume (uL)", y="Total Volume\nFlushed (uL)") -> (x+y=w3898:dbl)
            n2372 = local write "Total Volume\nFlushed (uL)"(w3898) -> ()
          }
          frame #1 {
            n2373 = Wait (ms)(milliseconds to wait=w3911) -> ()  [unwired: 1 out]
          }
          frame #2 {
            n2374 = call "Write to pump.vi"("string"="start", "VISA resource name"=w3912) -> ()  [unwired: 1 out]
          }
        }
        n2375 = local read "Chemyx Syringe Pump Serial Port"() -> (w3894:refnum<visa-resource-name>)
      }
      event "Sample Channel\nFlow": Value Change {
        n2376 = event-data() -> ()  [unwired: 7 out]
        n2377 = Select(t="irun" ("string"), s="Sample Channel\nFlow", f="stop" ("string")) -> (s? t:f=w3916:string)
        n2378 = Concatenate Strings(w3916, "\r") -> (w3919:string)
        n2379 = VISA Write(VISA resource name=w3914, write buffer=w3919) -> ()  [unwired: 1 in, 3 out]
      }
      event "Start Flow": Value Change {
        n2380 = event-data() -> ()  [unwired: 7 out]
        n2381 = local write "Sample Channel\nFlow"(TRUE ("Sample Channel\nFlow")) -> ()
        n2382 = local write "Start Flow"(FALSE ("Start Flow")) -> ()
        n2383 = Concatenate Strings("irun" ("string"), "\r") -> (w3925:string)
        n2384 = VISA Write(VISA resource name=w3921, write buffer=w3925) -> ()  [unwired: 1 in, 3 out]
      }
      event "Stop Flow": Value Change {
        w3927 = FALSE ("Stop Flow")
        n2385 = event-data() -> ()  [unwired: 7 out]
        n2386 = local write "Stop Flow"(w3927) -> ()
        n2387 = local write "Sample Channel\nFlow"(w3927) -> ()
        n2388 = Concatenate Strings("stop" ("string"), "\r") -> (w3930:string)
        n2389 = VISA Write(VISA resource name=w3928, write buffer=w3930) -> ()  [unwired: 1 in, 3 out]
      }
      event "Flow rate (uL/h)": Value Change {
        n2390 = event-data() -> ()  [unwired: 7 out]
        n2391 = Number To Decimal String(number="Flow rate (uL/h)") -> (decimal integer string=w3937:string)  [unwired: 1 in]
        n2392 = Concatenate Strings("irate  " ("string"), w3937, " u/h" ("string"), "\r") -> (w3936:string)
        n2393 = VISA Write(VISA resource name=w3933, write buffer=w3936) -> ()  [unwired: 1 in, 3 out]
      }
      event "Flush Sample": Value Change {
        n2394 = event-data() -> ()  [unwired: 7 out]
        n2395 = flat-sequence {
          tunnel: w3942 -> [w3970]
          tunnel: [w3950] -> w3941
          tunnel: [w3944] -> w3939
          tunnel: w3941 -> [w3974]
          tunnel: [w3974] -> w3940
          tunnel: w3939 -> [w3973]
          tunnel: w3940 -> [w3979]
          frame #0 {
            # "set paramaters (rate, volume) for flush, clear volume"
            n2396 = Number To Decimal String(number="Flush rate (uL/m)") -> (decimal integer string=w3966:string)  [unwired: 1 in]
            n2397 = Concatenate Strings("irate  " ("string"), w3966, " u/m" ("string"), "\r") -> (w3968:string)
            n2398 = VISA Write(VISA resource name=w3970, write buffer=w3968) -> (VISA resource name out=w3964:refnum<visa-resource-name>)  [unwired: 1 in, 2 out]
            n2399 = Reciprocal(x="Flush rate (uL/m)") -> (1/x=w3947:dbl)
            n2400 = Number To Decimal String(number="Volume (uL)") -> (decimal integer string=w3955:string)  [unwired: 1 in]
            n2401 = Multiply(x="Volume (uL)", y=w3947) -> (x*y=w3946:dbl)
            n2402 = Concatenate Strings("tvolume  " ("string"), w3955, " u" ("string"), "\r") -> (w3953:string)
            n2403 = Multiply(x=w3946, y=60000.0) -> (x*y=w3944:dbl)
            n2404 = VISA Write(VISA resource name=w3964, write buffer=w3953) -> (VISA resource name out=w3952:refnum<visa-resource-name>)  [unwired: 1 in, 2 out]
            n2405 = Concatenate Strings("cvolume" ("string"), "\r") -> (w3951:string)
            n2406 = VISA Write(VISA resource name=w3952, write buffer=w3951) -> (VISA resource name out=w3962:refnum<visa-resource-name>)  [unwired: 1 in, 2 out]
            n2407 = Concatenate Strings("irun" ("string"), "\r") -> (w3960:string)
            n2408 = VISA Write(VISA resource name=w3962, write buffer=w3960) -> (VISA resource name out=w3950:refnum<visa-resource-name>)  [unwired: 1 in, 2 out]
          }
          frame #1 {
            # "Have to wait until\nflow is done to reset\nrate"
            n2409 = Add(x=w3973, y=100.0) -> (x+y=w3972:dbl)
            n2410 = Wait (ms)(milliseconds to wait=w3972) -> ()  [unwired: 1 out]
          }
          frame #2 {
            # "reset flow rate to usual flow rate"
            n2411 = local read "Flow rate (uL/h)"() -> (w3985:dbl)
            n2412 = Number To Decimal String(number=w3985) -> (decimal integer string=w3983:string)  [unwired: 1 in]
            n2413 = Concatenate Strings("irate  " ("string"), w3983, " u/h" ("string"), "\r") -> (w3981:string)
            n2414 = VISA Write(VISA resource name=w3979, write buffer=w3981) -> (VISA resource name out=w3975:refnum<visa-resource-name>)  [unwired: 1 in, 2 out]
            n2415 = Concatenate Strings("cvolume" ("string"), "\r") -> (w3976:string)
            n2416 = VISA Write(VISA resource name=w3975, write buffer=w3976) -> ()  [unwired: 1 in, 3 out]
          }
        }
      }
      event "Flush Pump 3": Value Change {
        n2417 = event-data() -> ()  [unwired: 7 out]
        n2418 = flat-sequence {
          tunnel: w3986 -> [w3989]
          frame #0 {
            # "set paramaters (rate, volume) for flush, clear volume"
            n2419 = Number To Decimal String(number="Flush rate (uL/m) P3") -> (decimal integer string=w4011:string)  [unwired: 1 in]
            n2420 = local write "Inject Pump 3"(TRUE ("Inject Pump 3")) -> ()
            n2421 = Concatenate Strings("irate  " ("string"), w4011, " u/m" ("string"), "\r") -> (w4013:string)
            n2422 = VISA Write(VISA resource name=w3989, write buffer=w4013) -> (VISA resource name out=w4009:refnum<visa-resource-name>)  [unwired: 1 in, 2 out]
            n2423 = Reciprocal(x="Flush rate (uL/m) P3") -> (1/x=w3993:dbl)
            n2424 = Number To Decimal String(number="Volume (uL) P3") -> (decimal integer string=w4000:string)  [unwired: 1 in]
            n2425 = Multiply(x="Volume (uL) P3", y=w3993) -> (x*y=w3992:dbl)
            n2426 = Concatenate Strings("tvolume  " ("string"), w4000, " u" ("string"), "\r") -> (w3998:string)
            n2427 = Multiply(x=w3992, y=60.0) -> (x*y=→"HP3 Flush Time (s)":dbl)
            n2428 = VISA Write(VISA resource name=w4009, write buffer=w3998) -> (VISA resource name out=w3997:refnum<visa-resource-name>)  [unwired: 1 in, 2 out]
            n2429 = Concatenate Strings("cvolume" ("string"), "\r") -> (w3996:string)
            n2430 = VISA Write(VISA resource name=w3997, write buffer=w3996) -> (VISA resource name out=w4007:refnum<visa-resource-name>)  [unwired: 1 in, 2 out]
            n2431 = Concatenate Strings("irun" ("string"), "\r") -> (w4005:string)
            n2432 = VISA Write(VISA resource name=w4007, write buffer=w4005) -> ()  [unwired: 1 in, 3 out]
          }
          frame #1 {
            "Flushing P3" <- TRUE ("Flushing P3")
          }
        }
      }
      event "Flush Pump 1": Value Change {
        n2433 = event-data() -> ()  [unwired: 7 out]
        n2434 = flat-sequence {
          tunnel: [w4027] -> w4017
          tunnel: w4016 -> [w4020]
          tunnel: w4017 -> [_]
          frame #0 {
            # "set paramaters (rate, volume) for flush, clear volume"
            n2435 = local write "Inject Pump 1"(TRUE ("Inject Pump 1")) -> ()
            n2436 = Number To Decimal String(number="Flush rate (uL/m) P1") -> (decimal integer string=w4043:string)  [unwired: 1 in]
            n2437 = Concatenate Strings("irate  " ("string"), w4043, " u/m" ("string"), "\r") -> (w4045:string)
            n2438 = VISA Write(VISA resource name=w4020, write buffer=w4045) -> (VISA resource name out=w4041:refnum<visa-resource-name>)  [unwired: 1 in, 2 out]
            n2439 = Reciprocal(x="Flush rate (uL/m) P1") -> (1/x=w4024:dbl)
            n2440 = Number To Decimal String(number="Volume (uL) P1") -> (decimal integer string=w4032:string)  [unwired: 1 in]
            n2441 = Multiply(x="Volume (uL) P1", y=w4024) -> (x*y=w4023:dbl)
            n2442 = Concatenate Strings("tvolume  " ("string"), w4032, " u" ("string"), "\r") -> (w4030:string)
            n2443 = Multiply(x=w4023, y=60.0) -> (x*y=→"HP1 Flush Time (s)":dbl)
            n2444 = VISA Write(VISA resource name=w4041, write buffer=w4030) -> (VISA resource name out=w4029:refnum<visa-resource-name>)  [unwired: 1 in, 2 out]
            n2445 = Concatenate Strings("cvolume" ("string"), "\r") -> (w4028:string)
            n2446 = VISA Write(VISA resource name=w4029, write buffer=w4028) -> (VISA resource name out=w4039:refnum<visa-resource-name>)  [unwired: 1 in, 2 out]
            n2447 = Concatenate Strings("irun" ("string"), "\r") -> (w4037:string)
            n2448 = VISA Write(VISA resource name=w4039, write buffer=w4037) -> (VISA resource name out=w4027:refnum<visa-resource-name>)  [unwired: 1 in, 2 out]
          }
          frame #1 {
            "Flushing P1" <- TRUE ("Flushing P3")
          }
        }
      }
      event "Clear Volume": Value Change {
        n2449 = event-data() -> ()  [unwired: 7 out]
        n2450 = Concatenate Strings("cvolume" ("string"), "\r") -> (w4049:string)
        n2451 = VISA Write(VISA resource name=w4048, write buffer=w4049) -> ()  [unwired: 1 in, 3 out]
      }
      event "Clear Volume P3": Value Change {
        n2452 = event-data() -> ()  [unwired: 7 out]
        n2453 = Concatenate Strings("cvolume" ("string"), "\r") -> (w4055:string)
        n2454 = VISA Write(VISA resource name=w4054, write buffer=w4055) -> ()  [unwired: 1 in, 3 out]
        n2455 = local write "Clear Volume P3"(FALSE ("Clear Volume P3")) -> ()
      }
      event "Clear Volume P1": Value Change {
        n2456 = event-data() -> ()  [unwired: 7 out]
        n2457 = Concatenate Strings("cvolume" ("string"), "\r") -> (w4060:string)
        n2458 = local write "Clear Volume P1"(FALSE ("Clear Volume P1")) -> ()
        n2459 = VISA Write(VISA resource name=w4059, write buffer=w4060) -> ()  [unwired: 1 in, 3 out]
      }
      event "Display On P3": Value Change {
        n2460 = event-data() -> ()  [unwired: 7 out]
        n2461 = Select(t="dim 100", s="Display On P3", f="dim 0") -> (s? t:f=w4066:string)
        n2462 = Concatenate Strings(w4066, "\r") -> (w4068:string)
        n2463 = VISA Write(VISA resource name=w4063, write buffer=w4068) -> ()  [unwired: 1 in, 3 out]
      }
      event "Display On P1": Value Change {
        n2464 = event-data() -> ()  [unwired: 7 out]
        n2465 = Select(t="dim 100", s="Display On P1", f="dim 0") -> (s? t:f=w4073:string)
        n2466 = Concatenate Strings(w4073, "\r") -> (w4075:string)
        n2467 = VISA Write(VISA resource name=w4070, write buffer=w4075) -> ()  [unwired: 1 in, 3 out]
      }
      event "Retract Pump 3": Value Change {
        n2468 = event-data() -> ()  [unwired: 7 out]
        n2469 = local write "Retract Pump 3"(FALSE ("Retract Pump 3")) -> ()
        n2470 = case shown="True" "Retract Pump 3" {
          tunnel: w4077 -> [_ w4080]
          frame False {
          }
          frame True {
            n2471 = Number To Decimal String(number="Retract Rate (uL/m)") -> (decimal integer string=w4098:string)  [unwired: 1 in]
            n2472 = Concatenate Strings("wrate  " ("string"), w4098, " u/m" ("string"), "\r") -> (w4100:string)
            n2473 = VISA Write(VISA resource name=w4080, write buffer=w4100) -> (VISA resource name out=w4091:refnum<visa-resource-name>)  [unwired: 1 in, 2 out]
            n2474 = Number To Decimal String(number="Retract Vol 3 (uL)") -> (decimal integer string=w4093:string)  [unwired: 1 in]
            n2475 = Concatenate Strings("tvolume  " ("string"), w4093, " u" ("string"), "\r") -> (w4090:string)
            n2476 = VISA Write(VISA resource name=w4091, write buffer=w4090) -> (VISA resource name out=w4086:refnum<visa-resource-name>)  [unwired: 1 in, 2 out]
            n2477 = Concatenate Strings("cvolume" ("string"), "\r") -> (w4087:string)
            n2478 = VISA Write(VISA resource name=w4086, write buffer=w4087) -> (VISA resource name out=w4081:refnum<visa-resource-name>)  [unwired: 1 in, 2 out]
            n2479 = Concatenate Strings("wrun" ("string"), "\r") -> (w4082:string)
            n2480 = VISA Write(VISA resource name=w4081, write buffer=w4082) -> ()  [unwired: 1 in, 3 out]
          }
        }
      }
      event "Retract Pump 1": Value Change {
        n2481 = event-data() -> ()  [unwired: 7 out]
        n2482 = local write "Retract Pump 1"(FALSE ("Retract Pump 1")) -> ()
        n2483 = case shown="True" "Retract Pump 1" {
          tunnel: w4102 -> [_ w4107]
          frame False {
          }
          frame True {
            n2484 = local read "Retract Rate (uL/m)"() -> (w4105:dbl)
            n2485 = Number To Decimal String(number=w4105) -> (decimal integer string=w4123:string)  [unwired: 1 in]
            n2486 = Concatenate Strings("wrate  " ("string"), w4123, " u/m" ("string"), "\r") -> (w4125:string)
            n2487 = VISA Write(VISA resource name=w4107, write buffer=w4125) -> (VISA resource name out=w4117:refnum<visa-resource-name>)  [unwired: 1 in, 2 out]
            n2488 = Number To Decimal String(number="Retract Vol 1 (uL)") -> (decimal integer string=w4119:string)  [unwired: 1 in]
            n2489 = Concatenate Strings("tvolume  " ("string"), w4119, " u" ("string"), "\r") -> (w4116:string)
            n2490 = VISA Write(VISA resource name=w4117, write buffer=w4116) -> (VISA resource name out=w4113:refnum<visa-resource-name>)  [unwired: 1 in, 2 out]
            n2491 = Concatenate Strings("cvolume" ("string"), "\r") -> (w4114:string)
            n2492 = VISA Write(VISA resource name=w4113, write buffer=w4114) -> (VISA resource name out=w4108:refnum<visa-resource-name>)  [unwired: 1 in, 2 out]
            n2493 = Concatenate Strings("wrun" ("string"), "\r") -> (w4109:string)
            n2494 = VISA Write(VISA resource name=w4108, write buffer=w4109) -> ()  [unwired: 1 in, 3 out]
          }
        }
      }
      event "Flip Green Filter": Value Change {
        n2495 = event-data() -> ()  [unwired: 7 out]
        n2496 = Not(x="Flip Green Filter") -> (.not. x?=w4127:bool)
        n2497 = local write "Flip Green Filter"(w4127) -> ()
        n2498 = flat-sequence {
          tunnel: w4135 -> [w4140]
          tunnel: w4134 -> [w4139]
          tunnel: [w4137] -> w4132
          tunnel: [w4136] -> w4131
          tunnel: [w4142] -> w4130
          tunnel: w4132 -> [w4142]
          tunnel: [w4141] -> w4129
          tunnel: w4131 -> [w4141]
          tunnel: w4130 -> [w4146]
          tunnel: w4129 -> [w4145]
          tunnel: [w4144] -> w4133
          frame #0 {
            n2499 = xnode "Read/Write Control"("FPGA VI Reference In"=w4140, "error in"=w4139, "Green Filter Flipper"=TRUE) -> ("FPGA VI Reference Out"=w4137:T19, "error out"=w4136:errorcluster)
          }
          frame #1 {
            n2500 = Wait (ms)(milliseconds to wait=u32 100) -> ()  [unwired: 1 out]
          }
          frame #2 {
            n2501 = xnode "Read/Write Control"("FPGA VI Reference In"=w4146, "error in"=w4145, "Green Filter Flipper"=FALSE) -> ("error out"=w4144:errorcluster)  [unwired: 1 out]
          }
        }
      }
      event "Pump 1 contents", "Pump 3 contents": Value Change {
        n2502 = event-data() -> ()  [unwired: 7 out]
        n2503 = local read "Pump 1 contents"() -> (→"Pump 1 cont disp":string)
